vi "List Mode - Read Setting File Name.vi"(8 "error in (no error)":errorcluster, 11 "VISA resource name":refnum<visa-resource-name>) -> (0 "error out":errorcluster, 2 "File Name":string[](array[string]), 3 "VISA resource name out":refnum<visa-resource-name>)   [LabVIEW 2014, in "Associated Power Technologies 8500 Series.lvlib"]
doc: "Get from instrument the all setting file name on list mode."
uses:
  <instrlib>/Associated Power Technologies 8500 Series/Associated Power Technologies 8500 Series.lvlib
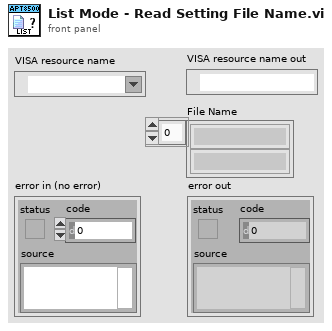
[diagram p1: front panel]
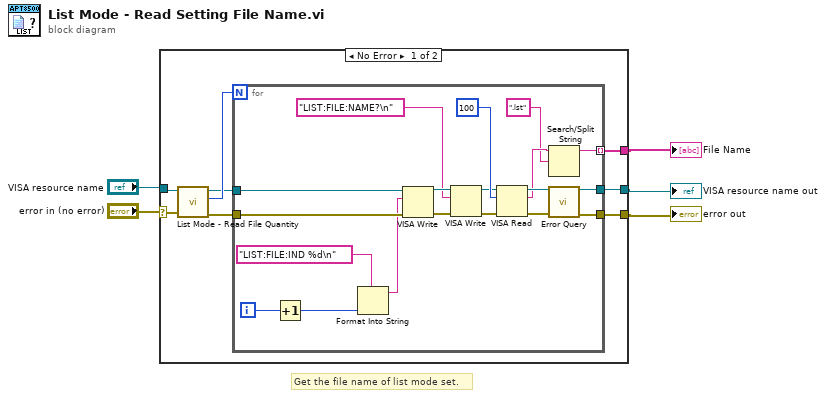
[diagram p0: block diagram]
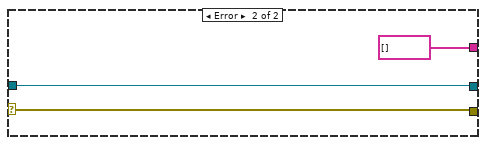
[diagram p2: hidden frame]
diagram:
  # "Get the file name of list mode set."
  n1 = case shown="No Error" "error in (no error)" {
    selector: "error in (no error)" -> [w9 w33]
    tunnel: "VISA resource name" -> [w10 w34]
    tunnel: [w13 string[] []] -> w1
    tunnel: [w12 w33] -> w2
    tunnel: [w11 w34] -> w3
    frame No Error {
      n2 = call <instrlib>:"List Mode - Read File Quantity.vi"("error in (no error)"=w9, "VISA resource name"=w10) -> ("error out"=w6:errorcluster, "Total File count"=w8:i32, "VISA resource name out"=w7:refnum<visa-resource-name>)  [unwired: 7 in]
      n3 = for {
        N: w8 -> [_]
        tunnel: w7 -> [w32]
        tunnel: w6 -> [w31]
        tunnel: [w22] -> w11
        tunnel: [w21] -> w12
        tunnel: [w18] -> w13 mode=indexing
        i -> [w15]
        n4 = Increment(x=w15) -> (x+1=w14:i32)
        n5 = Format Into String(format string="LIST:FILE:IND %d\n" ("write buffer"), w14) -> (resulting string=w16:string)  [unwired: 2 in, 1 out]
        n6 = VISA Write(VISA resource name=w32, write buffer=w16, error in (no error)=w31) -> (VISA resource name out=w25:refnum<visa-resource-name>, error out=w24:errorcluster)  [unwired: 1 out]
        n7 = VISA Write(VISA resource name=w25, write buffer="LIST:FILE:NAME?\n", error in (no error)=w24) -> (VISA resource name out=w28:refnum<visa-resource-name>, error out=w29:errorcluster)  [unwired: 1 out]
        n8 = VISA Read(VISA resource name=w28, byte count=u32 100 ("Bytes to Read"), error in (no error)=w29) -> (VISA resource name out=w27:refnum<visa-resource-name>, read buffer=w20:string, error out=w26:errorcluster)  [unwired: 1 out]
        n9 = Search/Split String(string=w20, search string/char (-)=".lst") -> (substring before match=w18:string)  [unwired: 1 in, 2 out]
        n10 = call <instrlib>:"Error Query.vi"("VISA resource name"=w27, "error in (no error)"=w26) -> ("VISA resource name out"=w22:refnum<visa-resource-name>, "error out"=w21:errorcluster)  [unwired: 10 in, 2 out]
      }
    }
    frame Error {
    }
  }
  "VISA resource name out" <- w3
  "error out" <- w2
  "File Name" <- w1
